vi "DigitalInOut.vi"(8 "error in (no error)":errorcluster, 9 "Existing Obj Name":string, 10 "Pin":string, 11 "mbed_LVLibrary.lvlib:mbed.lvclass":refnum<class "mbed.lvclass">) -> (0 "error out":errorcluster, 1 "Assigned Name":string, 3 "DigitalInOut.lvclass 2":refnum<class "DigitalInOut.lvclass">)   [LabVIEW 2011, in "mbed_LVLibrary.lvlib" / "DigitalInOut.lvclass"]
doc: "Creates a DigitalInOut object on mbed or ties to an existing digital input. Takes either a pin number as a string (eg \"p21\") or the name of an existign object on mbed"
uses:
  DigitalInOut.lvclass
  Transport Mechanisms/mbed/mbed.lvclass
  DigitalInOut.lvclass/DigitalInOut.ctl
  <vilib>/regexp/Match Regular Expression.xnode
panel:
  in  "DigitalInOut.lvclass":refnum<class "DigitalInOut.lvclass">
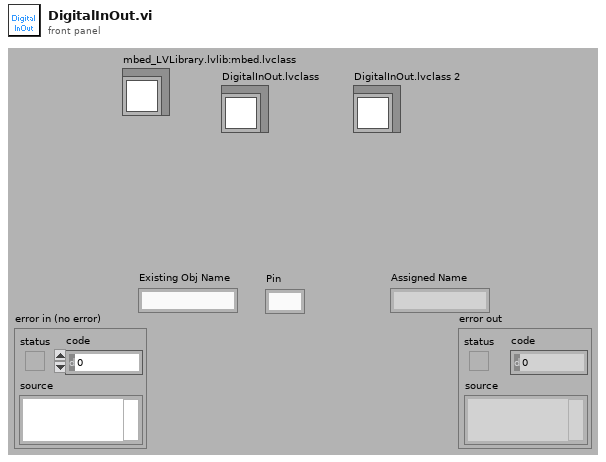
[diagram p1: front panel]
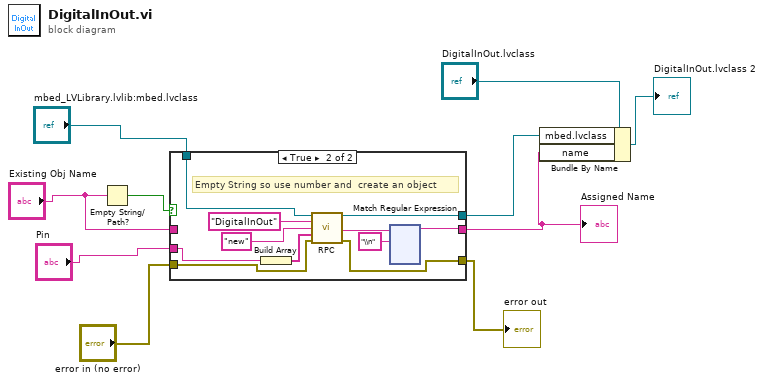
[diagram p0: block diagram]
diagram:
  n1 = Empty String/Path?(string/path="Existing Obj Name") -> (empty?=w8:bool)
  n2 = case shown="True" w8 {
    tunnel: "Existing Obj Name" -> [w13 _]
    tunnel: [w13 w20] -> w5
    tunnel: "mbed_LVLibrary.lvlib:mbed.lvclass" -> [w12 w24]
    tunnel: [w12 w21] -> w9
    tunnel: "Pin" -> [_ w16]
    tunnel: "error in (no error)" -> [w11 w15]
    tunnel: [w11 w14] -> w2
    frame False {
      # "String present so just set the class name"
    }
    frame True {
      # "Empty String so use number and  create an object"
      n3 = Build Array(w16) -> (w17:string[])
      n4 = call-dynamic "RPC.vi"("mbed in"=w24, "Name"="DigitalInOut", "method"="new", "Args"=w17, "error in (no error)"=w15) -> ("mbed out"=w21:refnum<class "mbed.lvclass">, "RPC Result"=w19:string, "error out"=w14:errorcluster)  [unwired: 8 in]
      n5 = xnode "Match Regular Expression"("input string"=w19, "regular expression"="\\n") -> ("before match"=w20:string)  [unwired: 4 in, 4 out]
    }
  }
  "Assigned Name" <- w5
  "error out" <- w2
  n6 = Bundle By Name(cluster="DigitalInOut.lvclass", "mbed.lvclass"=w9, "name"=w5) -> (→"DigitalInOut.lvclass 2":refnum<class "DigitalInOut.lvclass">)
